vi "Solution part 1.vi"(11 "data?":bool) -> ()   [LabVIEW 2020]
panel:
  out "result":i32
  out "bus ID":i32
  out "min wait time":i32
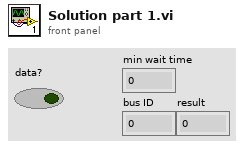
[diagram p1: front panel]
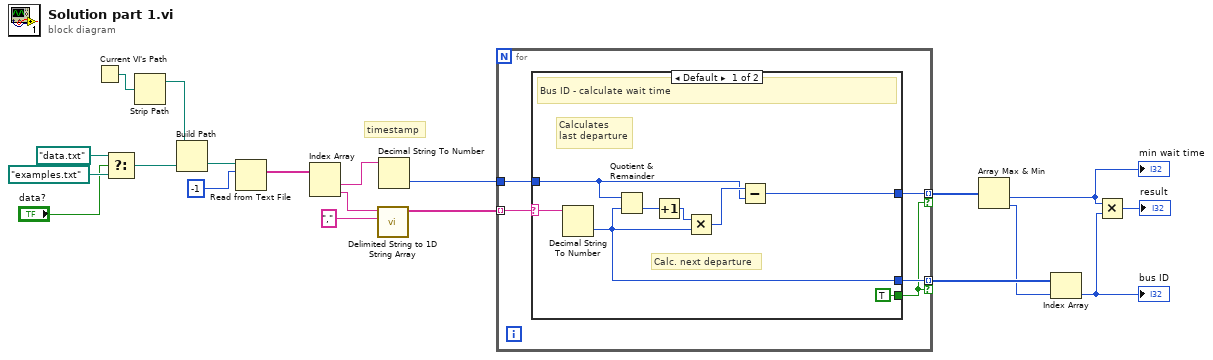
[diagram p0: block diagram]
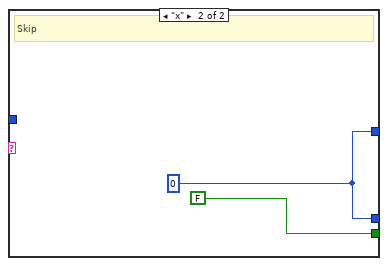
[diagram p2: hidden frame]
diagram:
  # "timestamp"
  n1 = Current VI's Path() -> (path=w17:path)
  n2 = Select(t=path "data.txt", s="data?", f=path "examples.txt") -> (s? t:f=w18:path)
  n3 = Strip Path(path=w17) -> (stripped path=w16:path)  [unwired: 1 out]
  n4 = Build Path(base path=w16, name or relative path=w18) -> (appended path=w15:path)
  n5 = Read from Text File(file (use dialog)=w15, count=-1) -> (text=w12:string[])  [unwired: 2 in, 3 out]
  n6 = Index Array(array=w12) -> (element #1=w11:string, element #2=w10:string)  [unwired: 2 in]
  n7 = call <vilib>:"Delimited String to 1D String Array.vi"("delimiter"=",", "delimited string"=w10) -> ("string array"=w8:string[])  [unwired: 9 in]
  n8 = Decimal String To Number(string=w11) -> (number=w7:i32)  [unwired: 2 in, 1 out]
  n9 = for {
    tunnel: w8 -> [w25] mode=indexing
    tunnel: w7 -> [w24]
    tunnel: [w23] -> w5 mode=indexing if=w21
    tunnel: [w22] -> w6 mode=indexing if=w21
    n10 = case shown="Default" w25 {
      selector: w25 -> [w33 _]
      tunnel: w24 -> [w27 _]
      tunnel: [w30 w34] -> w23
      tunnel: [TRUE FALSE] -> w21
      tunnel: [w26 w34] -> w22
      frame Default {
        # "Calc. next departure"
        # "Calculates \nlast departure"
        # "Bus ID - calculate wait time"
        n11 = Decimal String To Number(string=w33) -> (number=w30:i32)  [unwired: 2 in, 1 out]
        n12 = Quotient & Remainder(x=w27, y=w30) -> (floor(x/y)=w31:i32)  [unwired: 1 out]
        n13 = Increment(x=w31) -> (x+1=w29:i32)
        n14 = Multiply(x=w29, y=w30) -> (x*y=w28:i32)
        n15 = Subtract(x=w28, y=w27) -> (x-y=w26:i32)
      }
      frame "x" {
        w34 = 0
        # "Skip"
      }
    }
  }
  n16 = Array Max & Min(array=w6) -> (min value=w3:i32, min index (indices)=w4:i32)  [unwired: 2 out]
  "min wait time" <- w3
  n17 = Index Array(array=w5, index=w4) -> (element=w2:i32)
  "bus ID" <- w2
  n18 = Multiply(x=w3, y=w2) -> (x*y=→"result":i32)
